vi "Autoranging.vi"(7 "AUTORANGE":enum16{"DISABLED", "ENABLED"}(ring)=enum."ENABLED", 9 "ADC":i32, 10 "OVR":bool, 11 "RANGE":i32) -> (1 "RANGE HAS CHANGED":bool, 3 "NEW RANGE":i32, 4 "UNDERRANGE":bool, 5 "OVERRANGE":bool)   [LabVIEW 2012]
doc: "Suggests next higher or lower range,\nif ADC integer reading is over 19000 \nor below 1800. Does not change range."
panel:
  # "Autoranging.vi"
  # "If autorange=1 (enabled) and the ADC reading is either\nlower or higher than 1800 or 19000,  the next lower or higher\nmeasuring range is SUGGESTED and the \"range has changed\"\nindicator is set true. Please note that this VI does not change\nthe range, it only suggests a new range. Changing is made by\nsending new configuration to the bridge (remote must be enabled).\n\nIf range is already 2R or 2M, a lower or higher range cannot\nbe suggested. Then this VI only sets the underrange or overrange\nindicator.  ADC readings exceeding 19000 set the overrange indicator,\nwhereas the 7135 DVM subcircuit (=the ADC) sets its overrange flag\nwhen the input voltage exceeds 1.9999 volts (during overrange, the\nADC reading is exact zero).\n\nIf autoranging is disabled, the VI suggests the existing range. \n\nThe \"range has changed\" Boolean output can be used for  deciding,\nwhether to send the new configuration to the bridge or not."
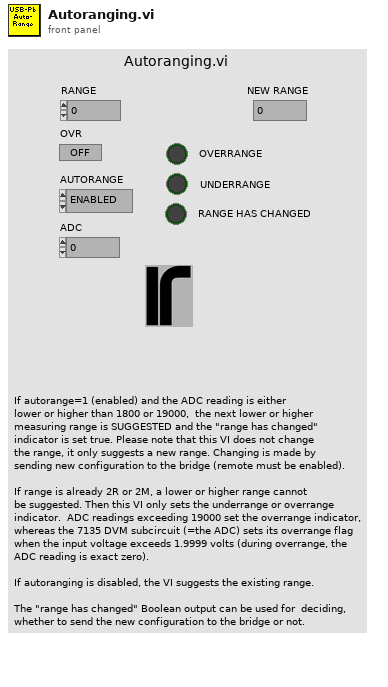
[diagram p1: front panel]
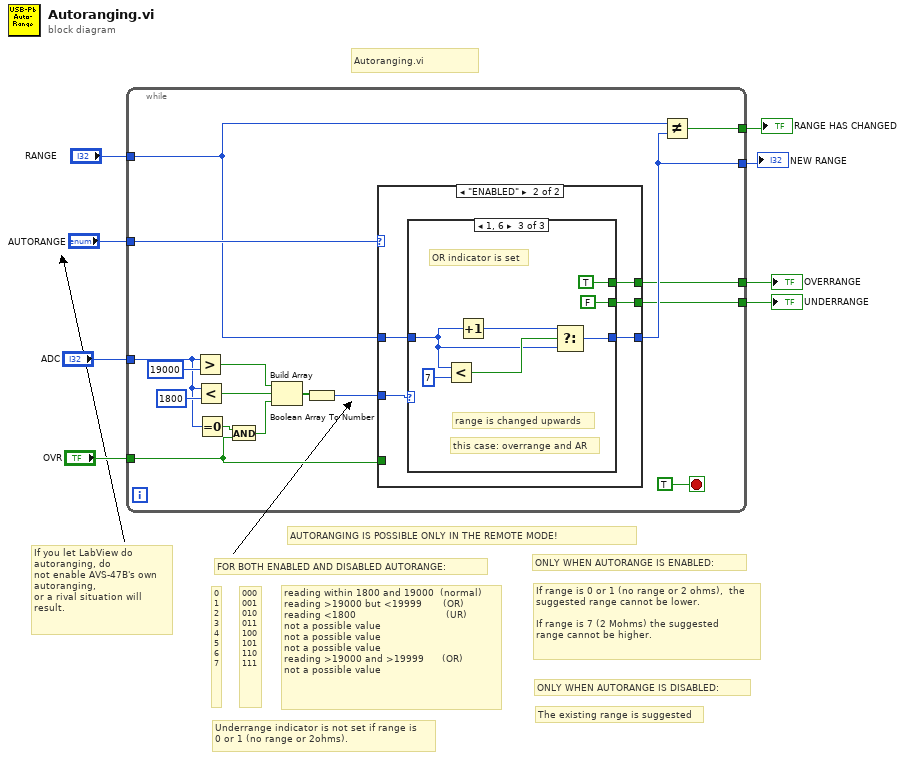
[diagram p0: block diagram]
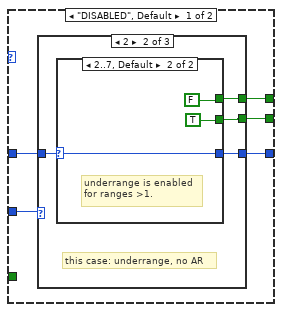
[diagram p2: hidden frame]
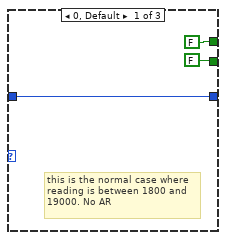
[diagram p3: hidden frame]
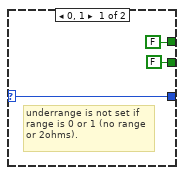
[diagram p4: hidden frame]
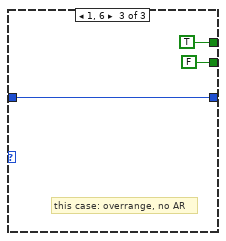
[diagram p5: hidden frame]
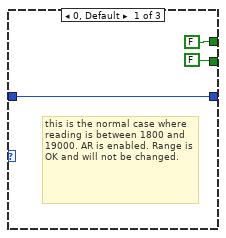
[diagram p6: hidden frame]
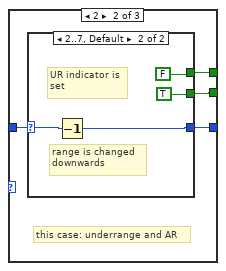
[diagram p7: hidden frame]
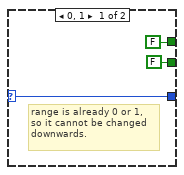
[diagram p8: hidden frame]
diagram:
  # "AUTORANGING IS POSSIBLE ONLY IN THE REMOTE MODE!"
  # "The existing range is suggested"
  # "ONLY WHEN AUTORANGE IS DISABLED:"
  # "If range is 0 or 1 (no range or 2 ohms),  the\nsuggested range cannot be lower.\n\nIf range is 7 (2 Mohms) the suggested\nrange cannot be higher."
  # "ONLY WHEN AUTORANGE IS ENABLED:"
  # "FOR BOTH ENABLED AND DISABLED AUTORANGE:"
  # "Underrange indicator is not set if range is \n0 or 1 (no range or 2ohms)."
  # "reading within 1800 and 19000  (normal)  reading >19000 but <19999       (OR)\nreading <1800                              (UR)\nnot a possible value\nnot a possible value\nnot a possible value\nreading >19000 and >19999      (OR)\nnot a possible value"
  # "0\n1\n2\n3\n4\n5\n6\n7"
  # "000\n001\n010\n011\n100\n101\n110\n111"
  # "If you let LabView do autoranging, do\nnot enable AVS-47B's own autoranging,\nor a rival situation will result."
  # "Autoranging.vi"
  n1 = while {
    tunnel: "AUTORANGE" -> [w24]
    tunnel: "ADC" -> [w11]
    tunnel: "OVR" -> [w10]
    tunnel: "RANGE" -> [w22]
    tunnel: [w23] -> w4
    tunnel: [w21] -> w3
    tunnel: [w20] -> w2
    tunnel: [w19] -> w1
    stop <- TRUE stop-if-true
    n2 = Greater?(x=w11, y=19000) -> (0:w15:bool)
    n3 = Less?(x=w11, y=1800) -> (x < y?=w14:bool)
    n4 = Equal To 0?(x=w11) -> (x = 0?=w16:bool)
    n5 = And(x=w16, y=w10) -> (x .and. y?=w13:bool)
    n6 = Build Array(w15, w14, w13) -> (w12:bool[])
    n7 = Boolean Array To Number(Boolean array=w12) -> (number=w9:u32)
    n8 = case shown="\"ENABLED\"" w24 {
      tunnel: [w29 w48] -> w20
      tunnel: [w28 w47] -> w19
      tunnel: w22 -> [w27 w50]
      tunnel: w10 -> [_ _]
      tunnel: [w30 w49] -> w23
      tunnel: w9 -> [w26 w51]
      frame "DISABLED", Default {
        n9 = case shown="2" w26 {
          tunnel: w27 -> [w33 w37 w44]
          tunnel: [w33 w34 w44] -> w30
          tunnel: [FALSE w36 TRUE] -> w29
          tunnel: [FALSE w35 FALSE] -> w28
          frame 0, Default {
            # "this is the normal case where\nreading is between 1800 and \n19000. No AR"
          }
          frame 2 {
            # "this case: underrange, no AR"
            n10 = case shown="2..7, Default" w37 {
              selector: w37 -> [w38 w43]
              tunnel: [FALSE FALSE] -> w36
              tunnel: [FALSE TRUE] -> w35
              tunnel: [w38 w43] -> w34
              frame 0, 1 {
                # "underrange is not set if\nrange is 0 or 1 (no range\nor 2ohms)."
              }
              frame 2..7, Default {
                # "underrange is enabled\nfor ranges >1."
              }
            }
          }
          frame 1, 6 {
            # "this case: overrange, no AR"
          }
        }
      }
      frame "ENABLED" {
        n11 = case shown="1, 6" w51 {
          tunnel: w50 -> [w54 w58 w67]
          tunnel: [w54 w55 w66] -> w49
          tunnel: [FALSE w57 TRUE] -> w48
          tunnel: [FALSE w56 FALSE] -> w47
          frame 0, Default {
            # "this is the normal case where\nreading is between 1800 and \n19000. AR is enabled. Range is OK and will not be changed."
          }
          frame 2 {
            # "this case: underrange and AR"
            n12 = case shown="2..7, Default" w58 {
              selector: w58 -> [w59 w63]
              tunnel: [FALSE FALSE] -> w57
              tunnel: [FALSE TRUE] -> w56
              tunnel: [w59 w62] -> w55
              frame 0, 1 {
                # "range is already 0 or 1, \nso it cannot be changed\ndownwards."
              }
              frame 2..7, Default {
                # "range is changed \ndownwards"
                # "UR indicator is\nset"
                n13 = Decrement(x=w63) -> (x-1=w62:i32)
              }
            }
          }
          frame 1, 6 {
            # "range is changed upwards"
            # "OR indicator is set"
            # "this case: overrange and AR"
            n14 = Less?(x=w67, y=7) -> (x < y?=w69:bool)
            n15 = Increment(x=w67) -> (x+1=w68:i32)
            n16 = Select(t=w68, s=w69, f=w67) -> (s? t:f=w66:i32)
          }
        }
      }
    }
    n17 = Not Equal?(x=w22, y=w23) -> (x != y?=w21:bool)
  }
  "OVERRANGE" <- w2
  "UNDERRANGE" <- w1
  "NEW RANGE" <- w4
  "RANGE HAS CHANGED" <- w3
